vi "Axis Control.vi"(10 "axis name":string="X", 11 "HasEncoder":bool) -> ()   [LabVIEW 2026]
uses:
  <instrlib>/A3200/Motion/EnableSingle.vi
  <instrlib>/A3200/Motion/AbortSingle.vi
  <instrlib>/A3200/Motion/FreerunSingle.vi
  <instrlib>/A3200/Bin/Aerotech.A3200.dll
panel:
  out "appended path":path
  out "name":string
  out "Position Feedback":string
  in  "Stop":bool
  in  "Go To":bool
  in  "Right":bool
  in  "Left":bool
  out "Encoder Position Feedback":string
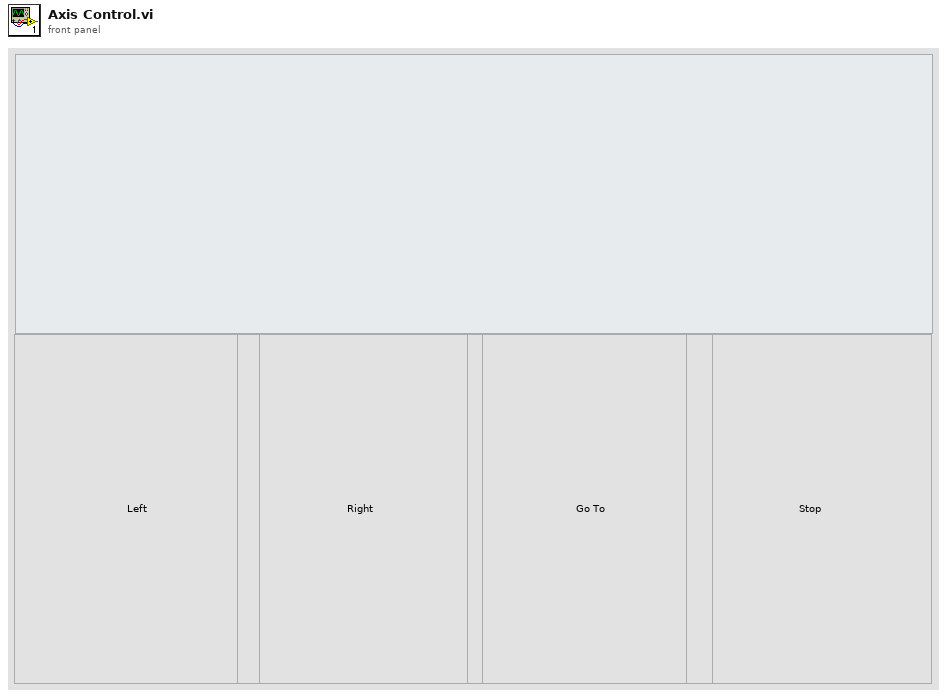
[diagram p1: front panel]
types:
  T1 = cluster{"new reference":refnum<k24>, "Event Callback":refnum<k27>, "ControllerDiagPacket":refnum<user-event>, "Event Registration Refnum":refnum<event-registration>}
  T2 = typedef "AxisDiagPacket.ctl" = cluster{"Axis Name":string, "Analog Input 0":dbl, "Analog Input 1":dbl, "Axis Fault (num)":i32, "Axis Fault (str)":string, "Axis Fault (bits)":cluster{"AmplifierFault":bool, "AmplifierTemperatureFault":bool, "CcwEndOfTravelLimitFault":bool, "CcwSoftwareLimitFault":bool, "CommunicationLostFault":bool, "CwEndOfTravelLimitFault":bool, "CwSoftwareLimitFault":bool, "EmergencyStopFault":bool, "EncoderFault":bool, "ExternalFault":bool, "FeedbackScalingFault":bool, "GantryMisalignFault ":bool, "HallSensorFault":bool, "InPositionTimeoutFault":bool, "MarkerSearchFault":bool, "MaxVelocityCommandFault":bool, "MissedInterruptFault":bool, "MotorTemperatureFault":bool, "None":bool, "OverCurrentFault":bool, "PositionErrorFault":bool, "PositionFeedbackFault":bool, "PowerSupplyFault":bool, "ProbeInputFault":bool, "SafeZoneFault":bool, "VelocityErrorFault":bool, "VelocityFeedbackFault":bool, "VoltageClampFault":bool, "InternalFault":bool}, "Axis Status (num)":i32, "Axis Status (str)":string, "Axis Status (bits)":cluster{"BacklashActive":bool, "CalibrationEnabled1D":bool, "CalibrationEnabled2D":bool, "CommandValid":bool, "DriveAbortPending":bool, "DrivePending":bool, "Enabling":bool, "GainMappingEnabled":bool, "GantryAligned":bool, "GantryRealigning":bool, "Homed":bool, "Homing":bool, "IFOVEnabled":bool, "JogGenerating":bool, "Jogging":bool, "JoystickControl":bool, "MasterSlaveControl":bool, "MotionBlocked":bool, "MotionClamped":bool, "MoveDone":bool, "None":bool, "NotVirtual":bool, "Profiling":bool, "Stability0":bool, "Stability1":bool, "TrajectoryFiltering":bool, "WaitDone":bool}, "Current Command":sgl, "Current Error":sgl, "Current Feedback":sgl, "Digital Inputs":i32, "Digital Outputs":i32, "Drive Status":i32, "Drive Status (str)":string, "Drive Status (bits)":cluster{"AccelerationPhase":bool, "AutofocusActive":bool, "BrakeOutput":bool, "CcwEndOfTravelLimitInput":bool, "CosineEncoderError":bool, "CurrentClamp":bool, "CwEndOfTravelLimitInput":bool, "DecelerationPhase":bool, "DualLoopActive":bool, "EmergencyStopInput":bool, "Enabled":bool, "EncoderClipping":bool, "GalvoCalibrationEnabled":bool, "GalvoPowerCorrection":bool, "HallAInput":bool, "HallBInput":bool, "HallCInput":bool, "HighResolutionMode":bool, "HomeLimitInput":bool, "InPosition":bool, "InPosition2":bool, "MarkerInput":bool, "MarkerLatch":bool, "MoveActive":bool, "NoMotorSupply":bool, "None":bool, "PowerLimiting":bool, "ProgrammingFlash":bool, "ProgrammingMXH":bool, "PSOHaltLatch":bool, "ServoControl":bool, "SineEncoderError":bool}, "Position Feedback Auxiliary":dbl, "Position Command":dbl, "Position Error":dbl, "Position Feedback":dbl, "Program Position Command":dbl, "Program Position Error":dbl, "Program Position Feedback":dbl, "Velocity Command":dbl, "Velocity Error":dbl, "Velocity Feedback":dbl}
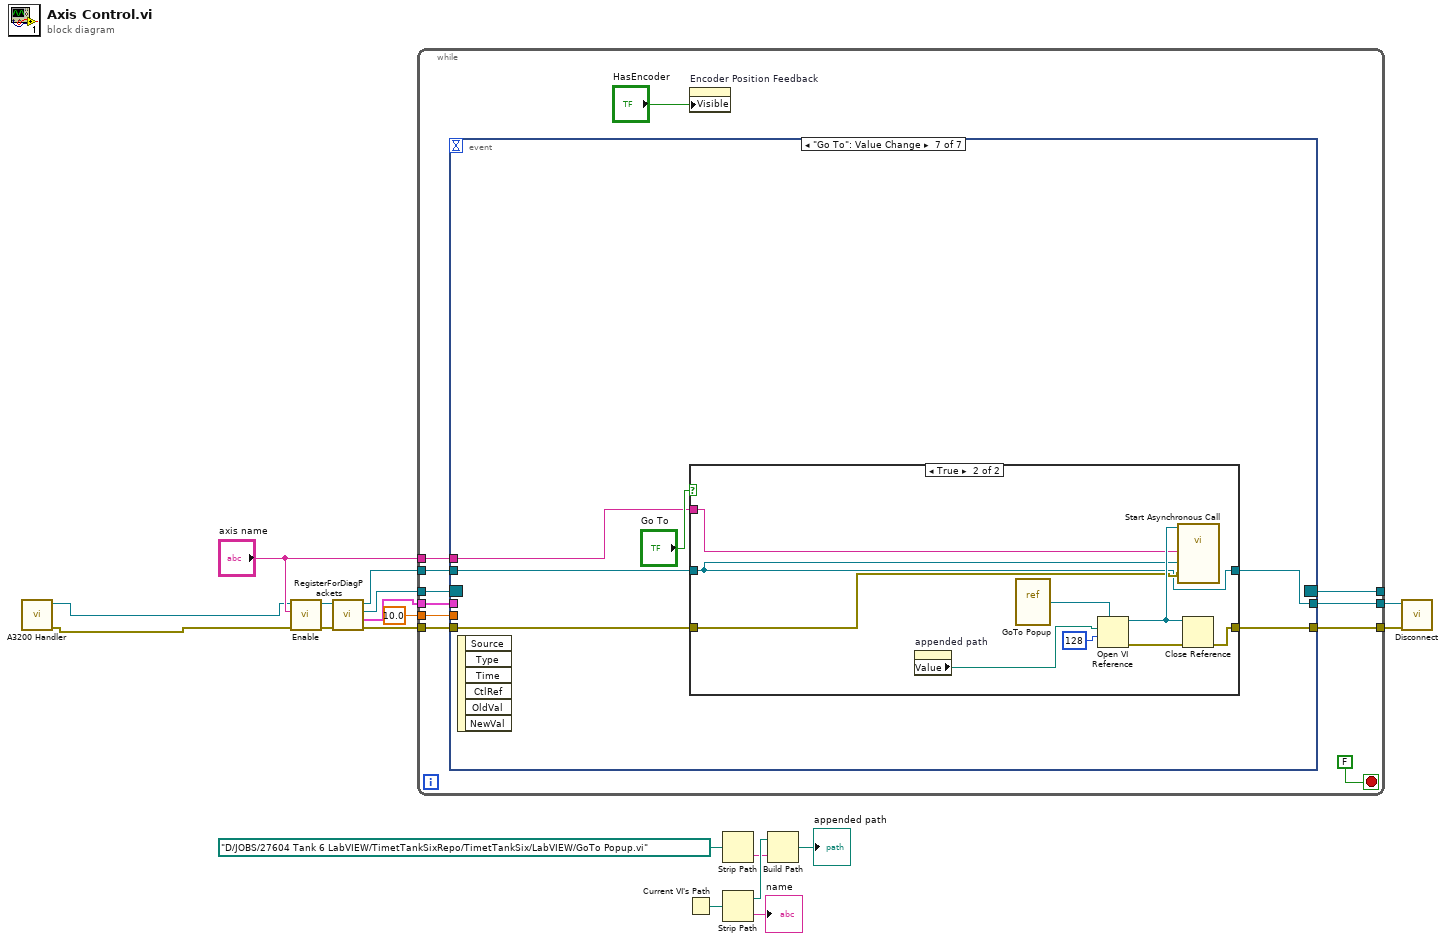
[diagram p0: block diagram]
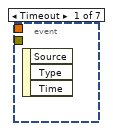
[diagram p2: hidden frame]
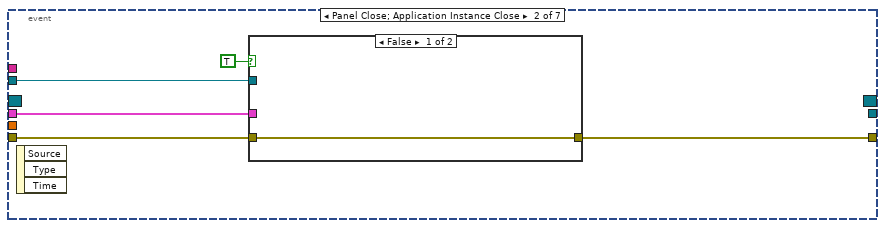
[diagram p3: hidden frame]
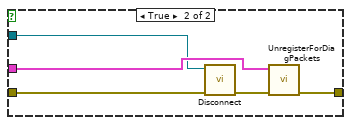
[diagram p4: hidden frame]
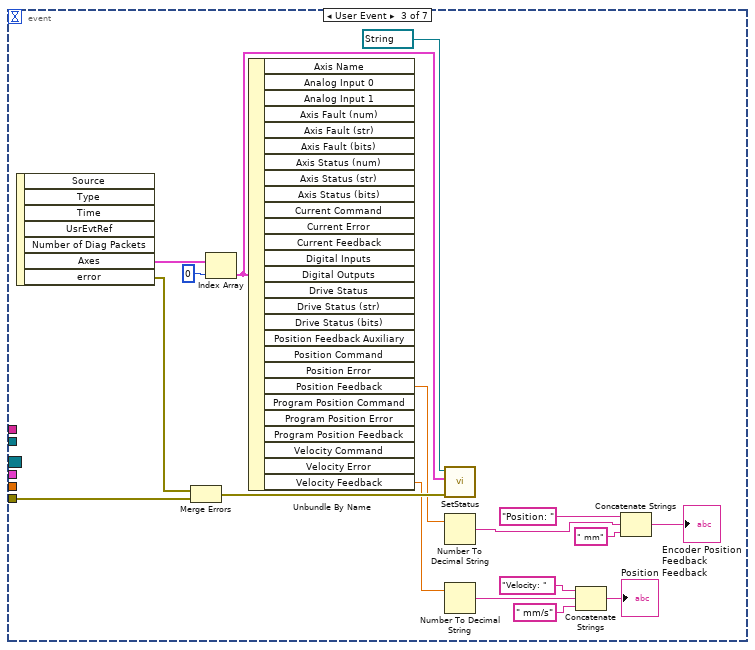
[diagram p5: hidden frame]
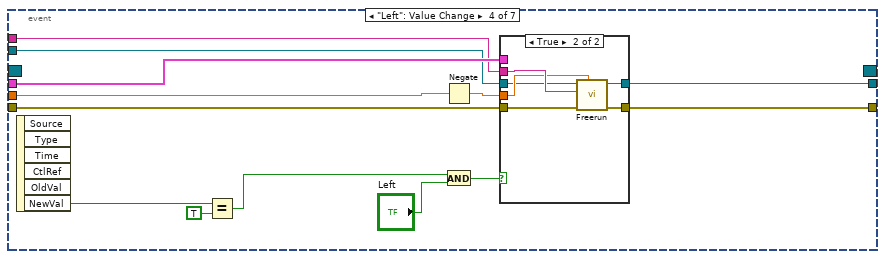
[diagram p6: hidden frame]
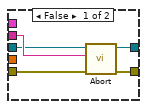
[diagram p7: hidden frame]
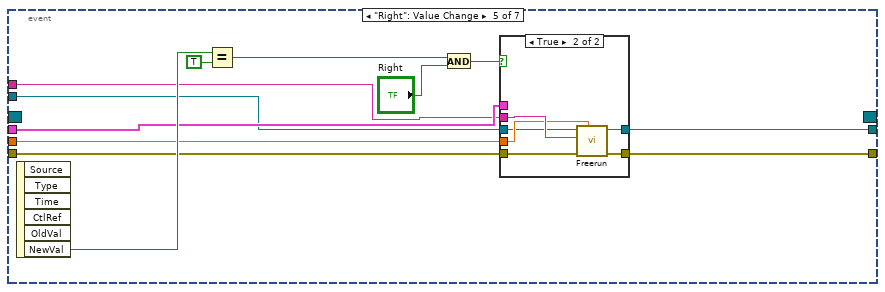
[diagram p8: hidden frame]
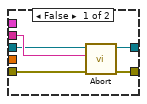
[diagram p9: hidden frame]
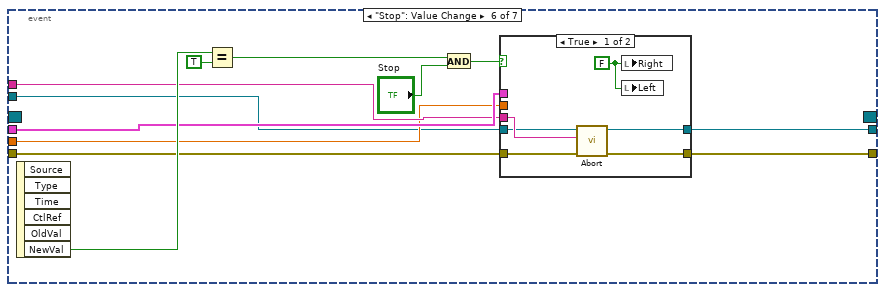
[diagram p10: hidden frame]
diagram:
  n1 = call "A3200 Handler.vi"() -> ("error out"=w2:errorcluster, "controller"=w1:refnum<k24>)  [unwired: 10 in]
  n2 = call-poly <instrlib>:"Enable.vi"("error in (no error)"=w2, "axis name"="axis name", "controller in"=w1) -> ("error out"=w16:errorcluster, "controller out"=w15:refnum<k24>)  [unwired: 7 in]
  n3 = call <instrlib>:"RegisterForDiagPackets.vi"("error in (no error)"=w16, "Controller in"=w15) -> ("error out"=w17:errorcluster, "Event Metadata"=w18:T1, "Event Registration Refnum"=w10:refnum<event-registration>, "Controller out"=w9:refnum<k24>)  [unwired: 5 in]
  n4 = while {
    tunnel: w18 -> [w28]
    tunnel: w17 -> [w27]
    tunnel: [w26] -> w12
    tunnel: [w25] -> _
    tunnel: "axis name" -> [w24]
    tunnel: 10.0 ("speed") -> [w23]
    tunnel: [w22] -> w11
    tunnel: w10 -> [w21]
    tunnel: w9 -> [w20]
    stop <- FALSE stop-if-true
    n5 = event shown="[6] \"Go To\": Value Change" {
      selector: w21 -> [_ _ _ _ _ _ _]
      dyn-events: [_ _ _ _ _ _ _] -> w25
      timeout: _ -> [_ _ _ _ _ _ _]
      tunnel: w28 -> [_ w34 _ w64 w88 w111 _]
      tunnel: w27 -> [_ w33 w55 w65 w89 w112 w128]
      tunnel: [_ w32 _ w62 w86 w109 w127] -> w26
      tunnel: w24 -> [_ _ _ w63 w87 w110 w129]
      tunnel: w23 -> [_ _ _ w61 w84 w108 _]
      tunnel: [_ _ _ w58 w82 w105 w126] -> w22
      tunnel: w20 -> [_ w30 _ w59 w83 w106 w125]
      event Timeout {
        n6 = event-data() -> ()  [unwired: 1 in, 3 out]
      }
      event Panel Close; Application Instance Close {
        n7 = event-data() -> ()  [unwired: 1 in, 3 out]
        n8 = case shown="False" TRUE {
          tunnel: w34 -> [_ w40]
          tunnel: w33 -> [w35 w39]
          tunnel: [w35 w37] -> w32
          tunnel: w30 -> [_ w36]
          frame False {
          }
          frame True {
            n9 = call <instrlib>:"Disconnect.vi"("error in (no error)"=w39, "controller"=w36) -> ("error out"=w38:errorcluster)  [unwired: 9 in]
            n10 = call <instrlib>:"UnregisterForDiagPackets.vi"("Event Metadata"=w40, "error in (no error)"=w38) -> ("error out"=w37:errorcluster)  [unwired: 8 in]
          }
        }
      }
      event User Event {
        n11 = event-data() -> ("Axes"=w53:T2[], "error"=w56:errorcluster)  [unwired: 1 in, 5 out]
        n12 = Merge Errors(w56, w55) -> (w54:errorcluster)
        n13 = Index Array(array=w53, index=0) -> (element=w52:T2)
        n14 = Unbundle By Name(w52) -> ("Position Feedback"=w43:dbl, "Velocity Feedback"=w51:dbl)  [unwired: 25 out]
        n15 = call <instrlib>:"SetStatus.vi"("error in (no error)"=w54, "AxisDiagPacket"=w52, "Status string"=refnum<vi> refnum) -> ()  [unwired: 8 in, 1 out]
        n16 = Number To Decimal String(number=w43) -> (decimal integer string=w46:string)  [unwired: 1 in]
        n17 = Number To Decimal String(number=w51) -> (decimal integer string=w50:string)  [unwired: 1 in]
        n18 = Concatenate Strings("Velocity: " ("string"), w50, " mm/s" ("string")) -> (→"Position Feedback":string)
        n19 = Concatenate Strings("Position: " ("string"), w46, " mm" ("string")) -> (→"Encoder Position Feedback":string)
      }
      event "Left": Value Change {
        n20 = event-data() -> ("NewVal"=w70:bool)  [unwired: 1 in, 5 out]
        n21 = Equal?(x=w70, y=TRUE) -> (x = y?=w67:bool)
        n22 = Negate(x=w61) -> (-x=w60:dbl)
        n23 = And(x=w67, y="Left") -> (x .and. y?=w68:bool)
        n24 = case shown="True" w68 {
          tunnel: w65 -> [w74 w80]
          tunnel: w64 -> [_ _]
          tunnel: w63 -> [w75 w81]
          tunnel: [w73 w79] -> w62
          tunnel: w60 -> [_ w78]
          tunnel: w59 -> [w72 w77]
          tunnel: [w71 w76] -> w58
          frame False {
            n25 = call-poly <instrlib>:"Abort.vi"("error in (no error)"=w74, "axis name? (all)"=w75, "controller in"=w72) -> ("error out"=w73:errorcluster, "controller out"=w71:refnum<k24>)  [unwired: 7 in]
          }
          frame True {
            n26 = call-poly <instrlib>:"Freerun.vi"("speed"=w78, "error in (no error)"=w80, "axis name"=w81, "controller in"=w77) -> ("error out"=w79:errorcluster, "controller out"=w76:refnum<k24>)  [unwired: 6 in]
          }
        }
      }
      event "Right": Value Change {
        n27 = event-data() -> ("NewVal"=w93:bool)  [unwired: 1 in, 5 out]
        n28 = Equal?(x=w93, y=TRUE) -> (x = y?=w90:bool)
        n29 = And(x=w90, y="Right") -> (x .and. y?=w91:bool)
        n30 = case shown="True" w91 {
          tunnel: w89 -> [w97 w103]
          tunnel: w88 -> [_ _]
          tunnel: w87 -> [w98 w104]
          tunnel: [w96 w102] -> w86
          tunnel: w84 -> [_ w101]
          tunnel: w83 -> [w95 w100]
          tunnel: [w94 w99] -> w82
          frame False {
            n31 = call-poly <instrlib>:"Abort.vi"("error in (no error)"=w97, "axis name? (all)"=w98, "controller in"=w95) -> ("error out"=w96:errorcluster, "controller out"=w94:refnum<k24>)  [unwired: 7 in]
          }
          frame True {
            n32 = call-poly <instrlib>:"Freerun.vi"("speed"=w101, "error in (no error)"=w103, "axis name"=w104, "controller in"=w100) -> ("error out"=w102:errorcluster, "controller out"=w99:refnum<k24>)  [unwired: 6 in]
          }
        }
      }
      event "Stop": Value Change {
        n33 = event-data() -> ("NewVal"=w116:bool)  [unwired: 1 in, 5 out]
        n34 = Equal?(x=w116, y=TRUE) -> (x = y?=w113:bool)
        n35 = And(x=w113, y="Stop") -> (x .and. y?=w114:bool)
        n36 = case shown="True" w114 {
          tunnel: w112 -> [w121 w124]
          tunnel: w111 -> [_ _]
          tunnel: w110 -> [w122 _]
          tunnel: [w120 w124] -> w109
          tunnel: w108 -> [_ _]
          tunnel: w106 -> [w118 w123]
          tunnel: [w117 w123] -> w105
          frame True {
            w119 = FALSE ("Left")
            n37 = call-poly <instrlib>:"Abort.vi"("error in (no error)"=w121, "axis name? (all)"=w122, "controller in"=w118) -> ("error out"=w120:errorcluster, "controller out"=w117:refnum<k24>)  [unwired: 7 in]
            n38 = local write "Right"(w119) -> ()
            n39 = local write "Left"(w119) -> ()
          }
          frame False {
          }
        }
      }
      event "Go To": Value Change {
        n40 = event-data() -> ()  [unwired: 1 in, 6 out]
        n41 = case shown="True" "Go To" {
          tunnel: w129 -> [_ w136]
          tunnel: w128 -> [w131 w137]
          tunnel: [w131 w140] -> w127
          tunnel: [w132 w135] -> w126
          tunnel: w125 -> [w132 w135]
          frame False {
          }
          frame True {
            n42 = property on="appended path" class="Path"() -> ("Value"=w133:path)  [unwired: 2 in, 2 out]
            n43 = vi-ref "GoTo Popup.vi"() -> (w134:refnum<vi>)
            n44 = Open VI Reference(type specifier VI Refnum (for type only)=w134, vi path=w133, options=128) -> (vi reference=w138:refnum<vi>, error out=w139:errorcluster)  [unwired: 3 in]
            n45 = call-by-ref "Start Asynchronous Call"(reference=w138, "error in (no error)"=w137, "controller in"=w135, "axis name"=w136) -> ()  [unwired: 1 in, 4 out]
            n46 = Close Reference(reference=w138, error in (no error)=w139) -> (error out=w140:errorcluster)
          }
        }
      }
    }
    n47 = property on="Encoder Position Feedback" class="Str"("Visible"="HasEncoder") -> ()  [unwired: 2 in, 2 out]
  }
  n48 = Current VI's Path() -> (path=w8:path)
  n49 = Strip Path(path=path "D:/JOBS/27604 Tank 6 LabVIEW/TimetTankSixRepo/TimetTankSix/LabVIEW/GoTo Popup.vi") -> (name=w3:string)  [unwired: 1 out]
  n50 = Strip Path(path=w8) -> (stripped path=w6:path, name=→"name":string)
  n51 = Build Path(base path=w6, name or relative path=w3) -> (appended path=→"appended path":path)
  n52 = call <instrlib>:"Disconnect.vi"("error in (no error)"=w12, "controller"=w11) -> ()  [unwired: 9 in, 1 out]
